vi "parseInclinationError.vi"(8 "error in (no error)":errorcluster, 10 "DynamicFrameParser":refnum<class "DynamicFrameParser.lvclass">, 11 "MIILC in":refnum<class "MIILC.lvclass">) -> (0 "error out":errorcluster, 3 "MIILC out":refnum<class "MIILC.lvclass">)   [LabVIEW 2016, in "RTMIILC.lvlib" / "MIILC.lvclass"]
uses:
  MIILC.lvclass
  Common_RT_Modbus/DynamicFrameParser/DynamicFrameParser.lvclass
  MIILC.lvclass/MIILC.ctl
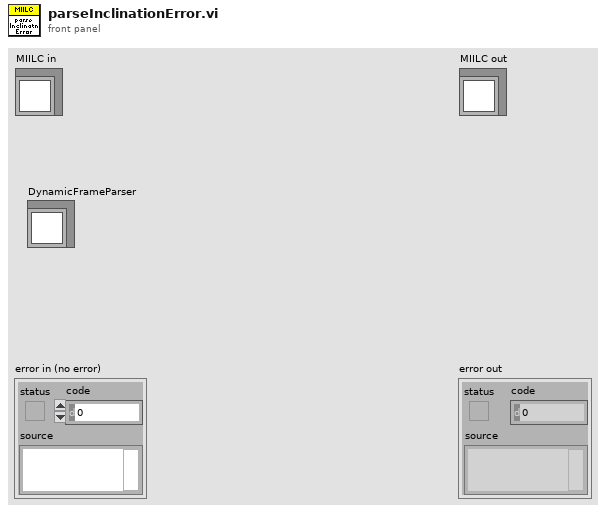
[diagram p1: front panel]
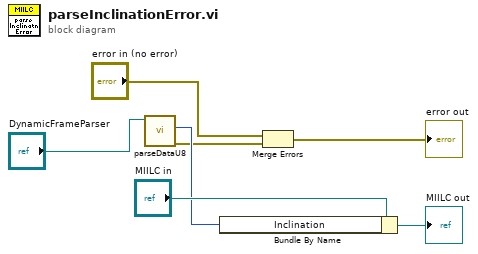
[diagram p0: block diagram]
diagram:
  n1 = call "parseDataU8.vi"("FrameParser in"="DynamicFrameParser") -> ("error out"=w1:errorcluster, "Data"=w2:u8)  [unwired: 8 in, 1 out]
  n2 = Bundle By Name(cluster="MIILC in", "Inclination"=w2) -> (→"MIILC out":refnum<class "MIILC.lvclass">)
  n3 = Merge Errors("error in (no error)", w1) -> (→"error out":errorcluster)
